vi "Esophageal_Datalogger_PlayButton.vi"(6 "Gain Value":dbl, 7 "Auto Exposure Status":bool, 8 "error in (no error)":errorcluster, 9 "Exposure Value":dbl, 10 "Auto Gain Status":bool, 11 "Log File In":refnum<file>) -> (0 "error out":errorcluster, 3 "Log File Out":refnum<file>)   [LabVIEW 2021]
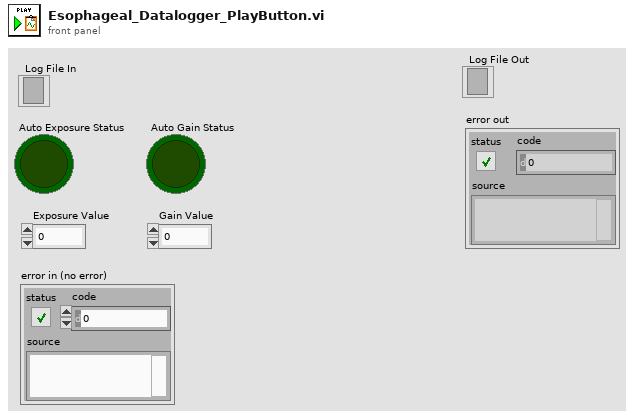
[diagram p1: front panel]
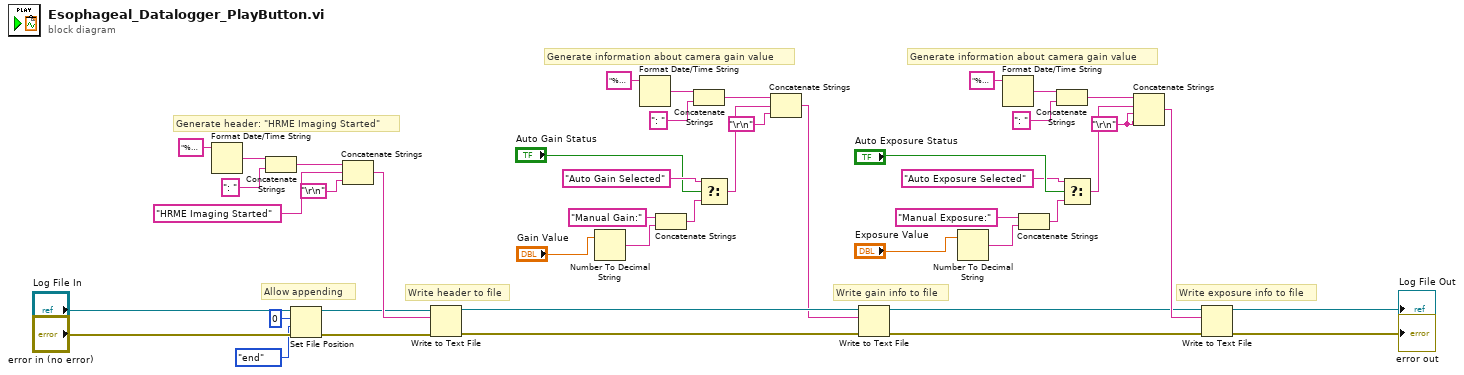
[diagram p0: block diagram]
diagram:
  w45 = "\r\n"
  # "Generate information about camera gain value"
  # "Generate information about camera gain value"
  # "Write gain info to file"
  # "Write header to file"
  # "Generate header: \"HRME Imaging Started\""
  # "Write exposure info to file"
  # "Allow appending"
  n1 = Format Date/Time String(time format string (%c)="%H%M%S%3u") -> (date/time string=w9:string)  [unwired: 2 in]
  n2 = Concatenate Strings(w9, ": " ("string")) -> (w11:string)
  n3 = Set File Position(offset (in bytes) (0)=i64 0, refnum="Log File In", from (0:start)=enum16{"start", "end", "current"}."end", error in="error in (no error)") -> (refnum out=w7:refnum<file>, error out=w15:errorcluster)
  n4 = Concatenate Strings(w11, "HRME Imaging Started" ("time format string (%c)"), "\r\n") -> (w14:string)
  n5 = Write to Text File(file (use dialog)=w7, text=w14, error in=w15) -> (refnum out=w22:refnum<file>, error out=w23:errorcluster)  [unwired: 1 in, 1 out]
  n6 = Number To Decimal String(number="Gain Value") -> (decimal integer string=w25:string)  [unwired: 1 in]
  n7 = Format Date/Time String(time format string (%c)="%H%M%S%3u") -> (date/time string=w19:string)  [unwired: 2 in]
  n8 = Concatenate Strings("Manual Gain:" ("string"), w25) -> (w27:string)
  n9 = Concatenate Strings(w19, ": " ("string")) -> (w17:string)
  n10 = Select(t="Auto Gain Selected" ("time format string (%c)"), s="Auto Gain Status", f=w27) -> (s? t:f=w28:string)
  n11 = Concatenate Strings(w17, w28, "\r\n") -> (w21:string)
  n12 = Write to Text File(file (use dialog)=w22, text=w21, error in=w23) -> (refnum out=w29:refnum<file>, error out=w31:errorcluster)  [unwired: 1 in, 1 out]
  n13 = Number To Decimal String(number="Exposure Value") -> (decimal integer string=w35:string)  [unwired: 1 in]
  n14 = Format Date/Time String(time format string (%c)="%H%M%S%3u") -> (date/time string=w38:string)  [unwired: 2 in]
  n15 = Concatenate Strings("Manual Exposure:" ("string"), w35) -> (w34:string)
  n16 = Concatenate Strings(w38, ": " ("string")) -> (w40:string)
  n17 = Select(t="Auto Exposure Selected" ("time format string (%c)"), s="Auto Exposure Status", f=w34) -> (s? t:f=w33:string)
  n18 = Concatenate Strings(w40, w33, w45, w45) -> (w42:string)
  n19 = Write to Text File(file (use dialog)=w29, text=w42, error in=w31) -> (refnum out=→"Log File Out":refnum<file>, error out=→"error out":errorcluster)  [unwired: 1 in, 1 out]
